vi "上位机.vi"() -> ()   [LabVIEW 2017]
uses:
  <vilib>/Instr/_visa.llb/VISA Configure Serial Port (Instr).vi
panel:
  out "警报灯":bool
  out "温度":dbl(graph)
  out "烟雾":dbl(graph)
  out "光强":dbl(graph)
  out "光强":dbl
  out "烟雾":dbl
  out "温度计":dbl(slide) scale=0.0..100.0
  in  "VISA配置":T1={"VISA resource name"="COM7", "baud rate (9600)"=2400, "data bits (8)"=8, "parity (0:none)"=0} {"parity (0:none)" items=["None", "Odd", "Even", "Mark", "Space"]; "data bits (8)" min=5 max=8 step=1}
  in  "停止":bool
  # "烟雾温度光强显示报警"
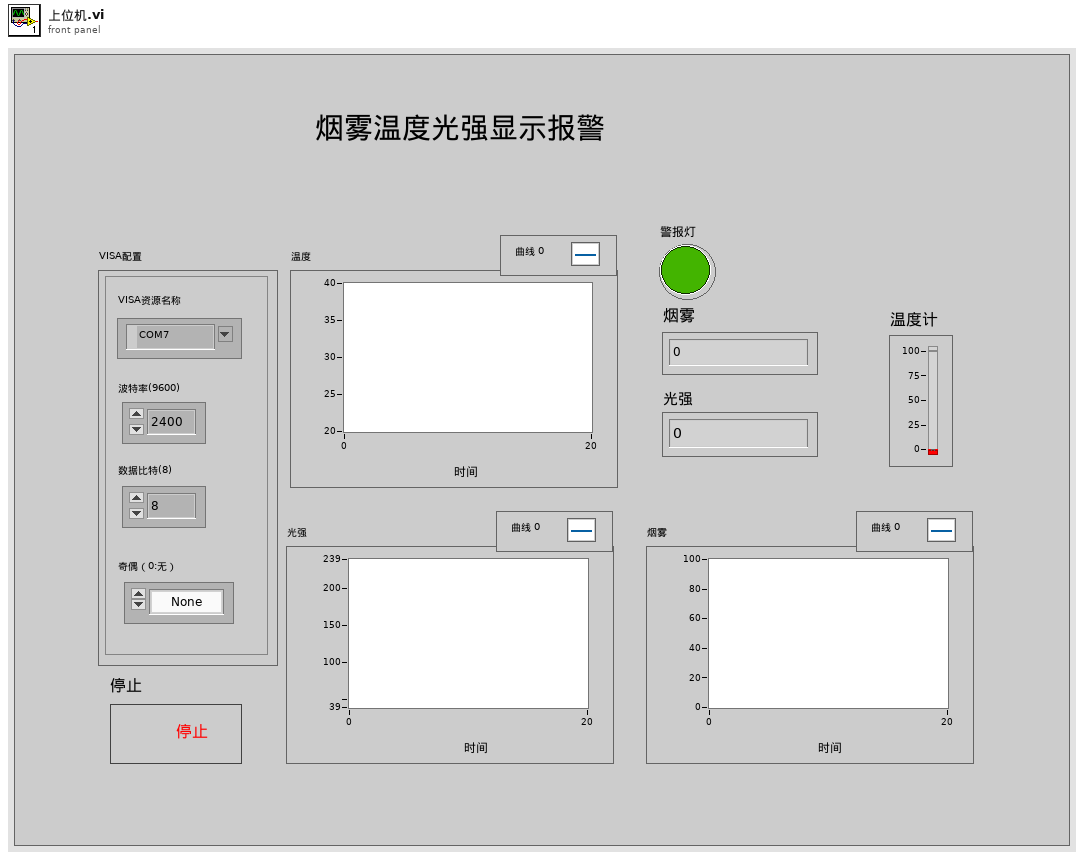
[diagram p1: front panel]
types:
  T1 = cluster{"VISA resource name":refnum<visa-resource-name>, "baud rate (9600)":u32, "data bits (8)":u16, "parity (0:none)":u16}
  T2 = enum16{"open", "replace", "create", "open or create", "replace or create", "replace or create with confirmation"}
  T3 = typedef "imagedata.ctl" = cluster{"image type":i32, "image depth":i32, "image":u8[], "mask":u8[], "colors":u32[], "Rectangle":cluster{"left":i16, "top":i16, "right":i16, "bottom":i16}}
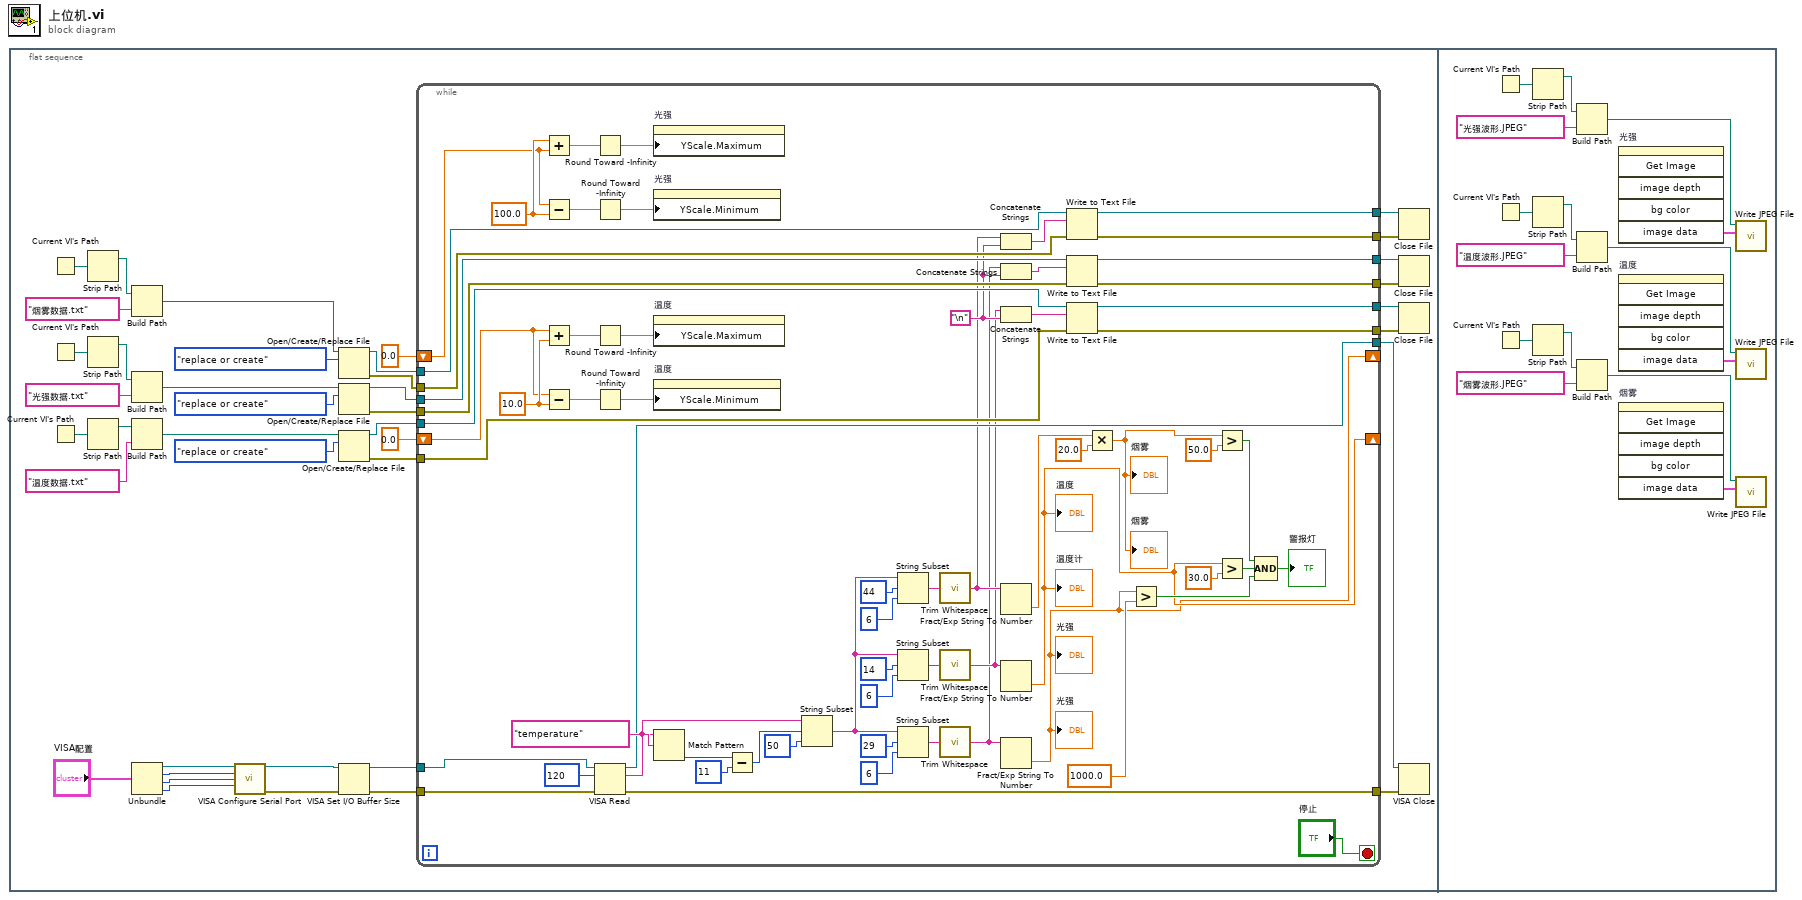
[diagram p0: block diagram]
diagram:
  n1 = flat-sequence {
    frame #0 {
      n2 = Current VI's Path() -> (path=w29:path)
      n3 = Current VI's Path() -> (path=w24:path)
      n4 = Current VI's Path() -> (path=w33:path)
      n5 = Strip Path(path=w29) -> (stripped path=w28:path)  [unwired: 1 out]
      n6 = Strip Path(path=w24) -> (stripped path=w9:path)  [unwired: 1 out]
      n7 = Strip Path(path=w33) -> (stripped path=w8:path)  [unwired: 1 out]
      n8 = Build Path(base path=w28, name or relative path="烟雾数据.txt" ("名称或相对路径")) -> (appended path=w26:path)
      n9 = Build Path(base path=w9, name or relative path="光强数据.txt" ("名称或相对路径")) -> (appended path=w22:path)
      n10 = Build Path(base path=w8, name or relative path="温度数据.txt" ("名称或相对路径")) -> (appended path=w31:path)
      n11 = Unbundle("VISA配置") -> ("VISA resource name"=w35:refnum<visa-resource-name>, "baud rate (9600)"=w39:u32, "data bits (8)"=w38:u16, "parity (0:none)"=w37:u16)
      n12 = call-poly "VISA Configure Serial Port"("VISA resource name"=w35, "baud rate (9600)"=w39, "data bits (8)"=w38, "parity (0:none)"=w37) -> ("VISA resource name out"=w3:refnum<visa-resource-name>, "error out"=w4:errorcluster)  [unwired: 10 in]
      n13 = Open/Create/Replace File(file path (use dialog)=w26, operation (0:open)=T2."replace or create" ("操作(0:open)")) -> (refnum out=w19:refnum<file>, error out=w18:errorcluster)  [unwired: 4 in, 1 out]
      n14 = Open/Create/Replace File(file path (use dialog)=w22, operation (0:open)=T2."replace or create" ("操作(0:open)")) -> (refnum out=w17:refnum<file>, error out=w16:errorcluster)  [unwired: 4 in, 1 out]
      n15 = Open/Create/Replace File(file path (use dialog)=w31, operation (0:open)=T2."replace or create" ("操作(0:open)")) -> (refnum out=w21:refnum<file>, error out=w20:errorcluster)  [unwired: 4 in, 1 out]
      n16 = VISA Set I/O Buffer Size(VISA resource name=w3, error in (no error)=w4) -> (VISA resource name out=w1:refnum<visa-resource-name>, error out=w2:errorcluster)  [unwired: 2 in]
      n17 = while {
        tunnel: [w62] -> w40
        tunnel: w21 -> [w91]
        tunnel: w20 -> [w90]
        tunnel: w19 -> [w89]
        tunnel: w18 -> [w88]
        tunnel: w17 -> [w87]
        tunnel: w16 -> [w86]
        tunnel: [w85] -> w15
        tunnel: [w84] -> w14
        tunnel: [w83] -> w13
        tunnel: [w82] -> w12
        tunnel: [w81] -> w11
        tunnel: [w80] -> w10
        shift-right: [w66] -> _
        shift-left: 0.0 -> [w50]
        shift-right: [w64] -> _
        shift-left: 0.0 -> [w49]
        tunnel: [w61] -> w5
        tunnel: w2 -> [w60]
        tunnel: w1 -> [w59]
        stop <- "停止" stop-if-true
        w58 = "\n"
        w63 = 100.0 ("y")
        w65 = 10.0 ("y")
        n18 = Add(x=w63, y=w49) -> (x+y=w48:dbl)
        n19 = Subtract(x=w49, y=w63) -> (x-y=w45:dbl)
        n20 = Add(x=w50, y=w65) -> (x+y=w44:dbl)
        n21 = Subtract(x=w50, y=w65) -> (x-y=w42:dbl)
        n22 = Round Toward -Infinity(1:w48) -> (0:w47:dbl)
        n23 = Round Toward -Infinity(1:w45) -> (0:w46:dbl)
        n24 = Round Toward -Infinity(1:w44) -> (0:w43:dbl)
        n25 = Round Toward -Infinity(1:w42) -> (0:w41:dbl)
        n26 = VISA Read(VISA resource name=w59, byte count=u32 120 ("大小(4096)"), error in (no error)=w60) -> (VISA resource name out=w61:refnum<visa-resource-name>, read buffer=w102:string, error out=w62:errorcluster)  [unwired: 1 out]
        n27 = property on="光强" class="WFChart (严格)"("YScale.Maximum"=w47) -> ()  [unwired: 2 in, 2 out]
        n28 = property on="光强" class="WFChart (严格)"("YScale.Minimum"=w46) -> ()  [unwired: 2 in, 2 out]
        n29 = property on="温度" class="WFChart (严格)"("YScale.Maximum"=w43) -> ()  [unwired: 2 in, 2 out]
        n30 = property on="温度" class="WFChart (严格)"("YScale.Minimum"=w41) -> ()  [unwired: 2 in, 2 out]
        n31 = Match Pattern(string=w102, regular expression="temperature") -> (offset past match=w103:i32)  [unwired: 1 in, 3 out]
        n32 = Subtract(x=w103, y=11) -> (x-y=w101:i32)
        n33 = String Subset(string=w102, offset (0)=w101, length (rest)=50 ("长度（剩余）")) -> (substring=w92:string)
        n34 = String Subset(string=w92, offset (0)=44 ("偏移量(0)"), length (rest)=6 ("长度（剩余）")) -> (substring=w77:string)
        n35 = String Subset(string=w92, offset (0)=14 ("偏移量(0)"), length (rest)=6 ("长度（剩余）")) -> (substring=w79:string)
        n36 = String Subset(string=w92, offset (0)=29 ("偏移量(0)"), length (rest)=6 ("长度（剩余）")) -> (substring=w75:string)
        n37 = call <vilib>:"Trim Whitespace.vi"("string"=w77) -> ("trimmed string"=w57:string)  [unwired: 1 in]
        n38 = call <vilib>:"Trim Whitespace.vi"("string"=w79) -> ("trimmed string"=w56:string)  [unwired: 1 in]
        n39 = call <vilib>:"Trim Whitespace.vi"("string"=w75) -> ("trimmed string"=w55:string)  [unwired: 1 in]
        n40 = Concatenate Strings(w57, w58) -> (w76:string)
        n41 = Concatenate Strings(w55, w58) -> (w74:string)
        n42 = Concatenate Strings(w56, w58) -> (w78:string)
        n43 = Fract/Exp String To Number(string=w57) -> (number=w53:dbl)  [unwired: 3 in, 1 out]
        n44 = Fract/Exp String To Number(string=w56) -> (number=w66:dbl)  [unwired: 3 in, 1 out]
        "温度计" <- w66
        "温度" <- w66
        n45 = Fract/Exp String To Number(string=w55) -> (number=w64:dbl)  [unwired: 3 in, 1 out]
        "光强" <- w64
        "光强" <- w64
        n46 = Write to Text File(file (use dialog)=w89, text=w76, error in=w88) -> (refnum out=w85:refnum<file>, error out=w84:errorcluster)  [unwired: 1 in, 1 out]
        n47 = Write to Text File(file (use dialog)=w87, text=w74, error in=w86) -> (refnum out=w81:refnum<file>, error out=w80:errorcluster)  [unwired: 1 in, 1 out]
        n48 = Write to Text File(file (use dialog)=w91, text=w78, error in=w90) -> (refnum out=w83:refnum<file>, error out=w82:errorcluster)  [unwired: 1 in, 1 out]
        n49 = Multiply(x=w53, y=20.0) -> (x*y=w51:dbl)
        "烟雾" <- w51
        "烟雾" <- w51
        n50 = Greater?(x=w64, y=1000.0) -> (0:w71:bool)
        n51 = Greater?(x=w51, y=50.0 ("x")) -> (0:w67:bool)
        n52 = Greater?(x=w66, y=30.0) -> (0:w69:bool)
        n53 = Compound Arithmetic op=AND ("复合运算")(w67, w69, w71) -> (→"警报灯":bool)
      }
      n54 = Close File(refnum=w15, error in=w14) -> ()  [unwired: 2 out]
      n55 = Close File(refnum=w11, error in=w10) -> ()  [unwired: 2 out]
      n56 = Close File(refnum=w13, error in=w12) -> ()  [unwired: 2 out]
      n57 = VISA Close(VISA resource name=w5, error in (no error)=w40) -> ()  [unwired: 1 out]
    }
    frame #1 {
      n58 = Current VI's Path() -> (path=w109:path)
      n59 = Current VI's Path() -> (path=w115:path)
      n60 = Current VI's Path() -> (path=w120:path)
      n61 = Strip Path(path=w109) -> (stripped path=w108:path)  [unwired: 1 out]
      n62 = Strip Path(path=w115) -> (stripped path=w114:path)  [unwired: 1 out]
      n63 = Strip Path(path=w120) -> (stripped path=w119:path)  [unwired: 1 out]
      n64 = Build Path(base path=w108, name or relative path="光强波形.JPEG" ("名称或相对路径")) -> (appended path=w106:path)
      n65 = Build Path(base path=w114, name or relative path="温度波形.JPEG" ("名称或相对路径")) -> (appended path=w112:path)
      n66 = Build Path(base path=w119, name or relative path="烟雾波形.JPEG" ("名称或相对路径")) -> (appended path=w117:path)
      n67 = invoke on="光强" class="WFChart (严格)" method="Get Image"() -> ("image data"=w110:T3)  [unwired: 6 in, 5 out]
      n68 = invoke on="温度" class="WFChart (严格)" method="Get Image"() -> ("image data"=w111:T3)  [unwired: 6 in, 5 out]
      n69 = invoke on="烟雾" class="WFChart (严格)" method="Get Image"() -> ("image data"=w116:T3)  [unwired: 6 in, 5 out]
      n70 = call <vilib>:"Write JPEG File.vi"("image data"=w110, "path to JPEG file"=w106) -> ()  [unwired: 8 in, 2 out]
      n71 = call <vilib>:"Write JPEG File.vi"("image data"=w111, "path to JPEG file"=w112) -> ()  [unwired: 8 in, 2 out]
      n72 = call <vilib>:"Write JPEG File.vi"("image data"=w116, "path to JPEG file"=w117) -> ()  [unwired: 8 in, 2 out]
    }
  }
